vi "DSF.Shared.Configuration.Framework.Get Plugin Configurations.vi"(11 "Framework Configuration in":refnum<class "DSF.Shared.Configuration.Framework.lvclass">) -> (2 "Plugin Configurations":refnum<class "DSF.Shared.Configuration.Plugin.lvclass">[](array[class]), 3 "Framework Configuration out":refnum<class "DSF.Shared.Configuration.Framework.lvclass">)   [LabVIEW 2017, in "DSF.Engine.lvlib" / "DSF.Shared.Configuration.Framework.lvclass"]
uses:
  DSF.Shared.Configuration.Framework.lvclass
  Plugin/DSF.Shared.Configuration.Plugin.lvclass
  DSF.Shared.Configuration.Framework.lvclass/DSF.Shared.Configuration.Framework.ctl
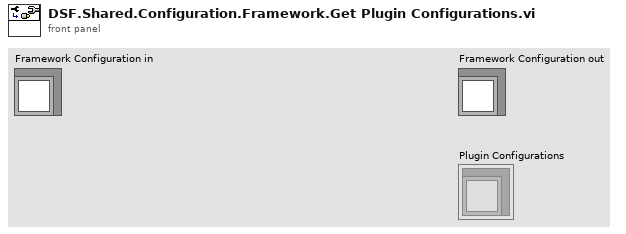
[diagram p1: front panel]
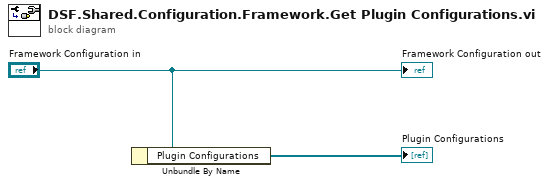
[diagram p0: block diagram]
diagram:
  n1 = Unbundle By Name("Framework Configuration in") -> ("Plugin Configurations"=→"Plugin Configurations":refnum<class "DSF.Shared.Configuration.Plugin.lvclass">[])
  "Framework Configuration out" <- "Framework Configuration in"
